vi "CRYFlatten waveform.vi"(11 "Waveform Cluster":T1={"Waveform"={"X0"=0.0, "dX"=0.0, "Y"=[]}, "X data"=1, "Y data"=1, "Y axis"=1, "X unit"="s", "Y unit"="V", "Y dB ref"=1.0, "display Y"=TRUE, "display X"=TRUE, "Overload?"=FALSE, "Test Info"="", "Step No."=0, "Name"="", "protected"=FALSE, "Sqc history"=[], "Signal Channel ID"=0, "Plot Settings"={"Color"=0, "Interpolation"=0, "Point Style"=0, "Line Style"=0, "Point Color"=0, "Line Width"=0, "Bar Plot Style"=0, "Fill To"=0}, "AutoProtect"=FALSE} {"Y dB ref" format="%.1f"; "Y axis" items=["Log", "Lin"]; "Y data" items=["dB", "Lin"]; "X data" items=["dB", "Lin"]}) -> (3 "Flatten Waveform":string)   [LabVIEW 2013]
uses:
  Typedef Control/CRYWaveform Cluster.ctl
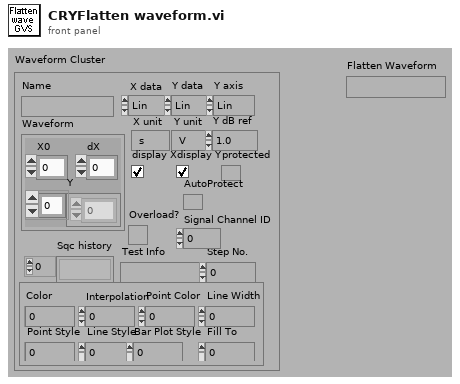
[diagram p1: front panel]
types:
  T1 = typedef "CRYWaveform Cluster.ctl" = cluster{"Waveform":cluster{"X0":dbl, "dX":dbl, "Y":sgl[]}, "X data":u16, "Y data":u16, "Y axis":u16, "X unit":string, "Y unit":string, "Y dB ref":dbl, "display Y":bool, "display X":bool, "Overload?":bool, "Test Info":string, "Step No.":i32, "Name":string, "protected":bool, "Sqc history":string[], "Signal Channel ID":i32, "Plot Settings":cluster{"Color":u32, "Interpolation":u8, "Point Style":u8, "Line Style":u8, "Point Color":u32, "Line Width":u8, "Bar Plot Style":u8, "Fill To":i16}, "AutoProtect":bool}
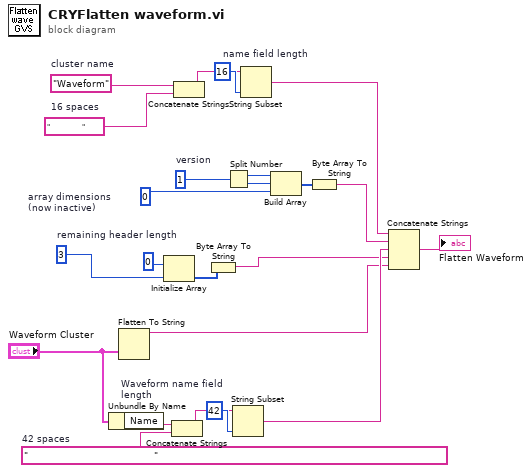
[diagram p0: block diagram]
diagram:
  w2 = "                                          "  # 42 spaces
  w8 = 42  # Waveform name field length
  w10 = u8 0  # array dimensions (now inactive)
  w13 = 16  # name field length
  w14 = "                "  # 16 spaces
  w15 = "Waveform"  # cluster name
  w19 = 3  # remaining header length
  w23 = u16 1  # version
  n1 = Unbundle By Name("Waveform Cluster") -> ("Name"=w9:string)
  n2 = Flatten To String(anything="Waveform Cluster") -> (data string=w4:string)  [unwired: 3 in, 2 out]
  n3 = Initialize Array(u8 0, w19) -> (w6:u8[])
  n4 = Concatenate Strings(w9, w2) -> (w7:string)
  n5 = Concatenate Strings(w15, w14) -> (w12:string)
  n6 = Byte Array To String(unsigned byte array=w6) -> (string=w3:string)
  n7 = Split Number(x=w23) -> (hi(x)=w22:u8, lo(x)=w21:u8)
  n8 = String Subset(string=w7, length (rest)=w8) -> (substring=w5:string)  [unwired: 1 in]
  n9 = String Subset(string=w12, length (rest)=w13) -> (substring=w11:string)  [unwired: 1 in]
  n10 = Build Array(w22, w21, w10) -> (w18:u8[])
  n11 = Byte Array To String(unsigned byte array=w18) -> (string=w16:string)
  n12 = Concatenate Strings(w11, w16, w5, w3, w4) -> (→"Flatten Waveform":string)
